vi "Strip EthernetFrame (UDP).vi"(11 "UDP Frame In":u8[](array[numeric]) format="%.0x") -> (2 "UDP header":T1, 3 "Payload":u8[](array[numeric]) format="%.0x")   [LabVIEW 2020, in "EthFrameManagement.lvlib"]
doc: "Obtain an UDP Frame from an Ethernet Frame."
uses:
  EthFrameManagement.lvlib
  controls/UDPFrame_type.ctl
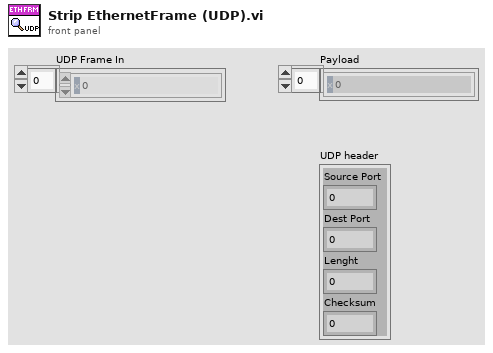
[diagram p1: front panel]
types:
  T1 = typedef "EthFrameManagement.lvlib/UDPFrame_type.ctl" = cluster{"Source Port":u16, "Dest Port":u16, "Lenght":u16, "Checksum":u16}
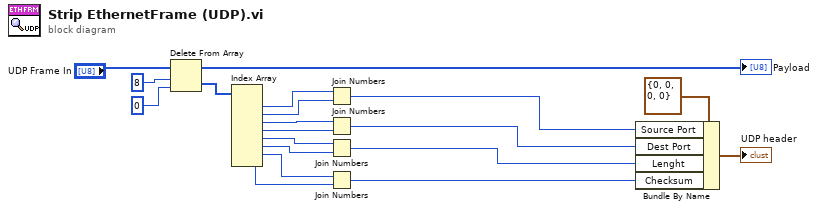
[diagram p0: block diagram]
diagram:
  n1 = Delete From Array(array="UDP Frame In", length=8, index=0) -> (deleted portion=w14:u8[], array with subset deleted=→"Payload":u8[])
  n2 = Index Array(array=w14) -> (element #1=w8:u8, element #2=w7:u8, element #3=w6:u8, element #4=w5:u8, element #5=w4:u8, element #6=w3:u8, element #7=w2:u8, element #8=w1:u8)  [unwired: 8 in]
  n3 = Join Numbers(hi=w8, lo=w7) -> ((hi.lo)=w13:u16)
  n4 = Join Numbers(hi=w6, lo=w5) -> ((hi.lo)=w12:u16)
  n5 = Join Numbers(hi=w4, lo=w3) -> ((hi.lo)=w11:u16)
  n6 = Join Numbers(hi=w2, lo=w1) -> ((hi.lo)=w10:u16)
  n7 = Bundle By Name(cluster=T1 {"Source Port"=0, "Dest Port"=0, "Lenght"=0, "Checksum"=0} ("IP Header"), "Source Port"=w13, "Dest Port"=w12, "Lenght"=w11, "Checksum"=w10) -> (→"UDP header":T1)
